vi "System Log.vi"(6 "VIs Hierarchy":i32, 8 "error in (no error)":errorcluster, 10 "Text to log":string, 11 "Object in":refnum<class>) -> (0 "error out":errorcluster)   [LabVIEW 2026, in "TALOS.lvlib"]
doc: "Log the text in the system log.\nVIs Hierarchy is used for selecting the name of which VI above this will be used in the log."
uses:
  TALOS.lvlib
  Ancestor/Ancestor/Ancestor.lvclass
  Ancestor/Ancestor/Ancestor.lvclass/Ancestor.ctl
  Classes/Log/Log.lvclass/Log.ctl
  Ancestor/Ancestor/Read ID.vi
  <vilib>/AdvancedString/Delimited String to 1D String Array.vi
  <vilib>/AdvancedString/Delimited String to 1D String Array (string).vi
  Classes/Log/Write.vi
  Generate Error.vi
  Date n Time.vi
  FGV/Error Memory/Get Error Description.vi
  Get PC name.vi
  <vilib>/Utility/error.llb/Clear Errors.vi
  FGV/Error Memory/Error Memory Core.vi
  Circus Root Path.vi
  FGV/Error Memory/Error Crt Lvl checker.vi
  FGV/Error Memory/Error Memory Core.vi/40c8088d-b597-4017-91af-faa98e00292e.vi
  FGV/Error Memory/Error Memory Core.vi/d4a3ab98-063c-4e44-b43d-fbdcfe6c2be2.vi
  <vilib>/Utility/LVClass/Get LV Class Name.vi
  Classes/Log/Rotate.vi
  Global Memory.vi
  Is in Packed Library.vi
  TALOS Root path.vi
  Read CSV worksheet.vi
  Global Constants.vi
  <vilib>/Utility/error.llb/General Error Handler.vi
  <vilib>/Comparison/Equal/Equal Functor/Equal Functor.lvclass
  Classes/Log/Log.lvclass
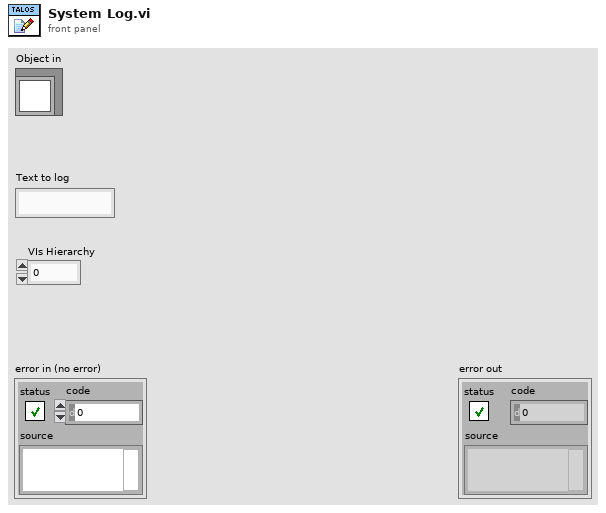
[diagram p1: front panel]
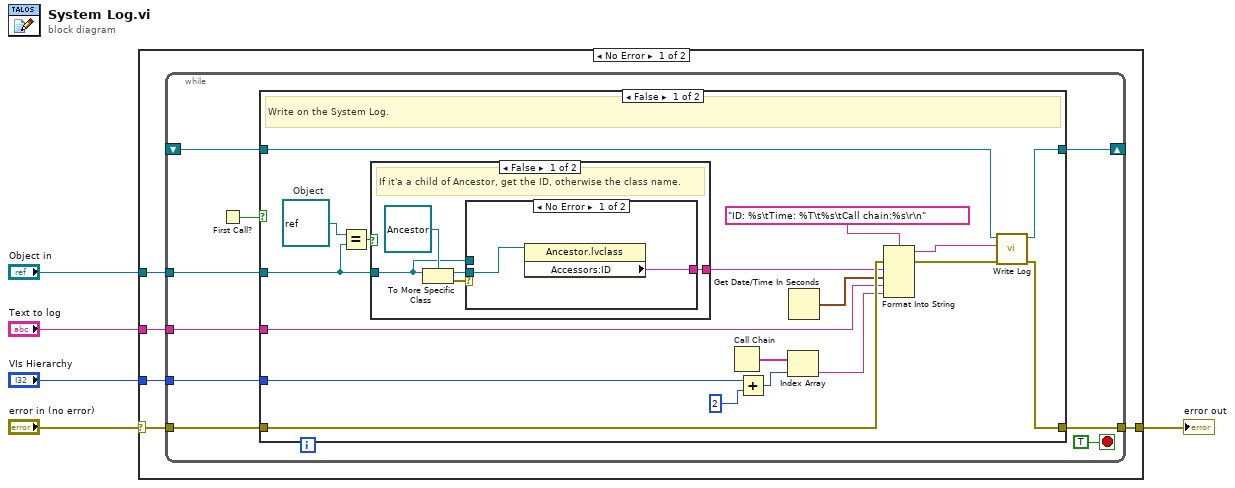
[diagram p0: block diagram]
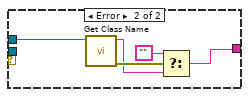
[diagram p2: hidden frame]
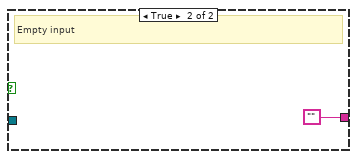
[diagram p3: hidden frame]
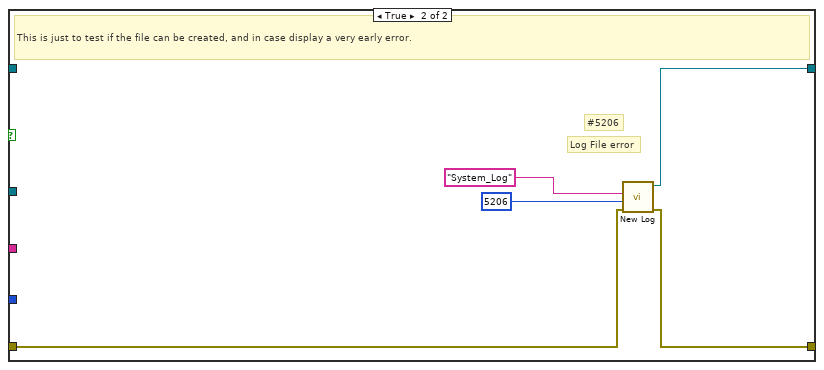
[diagram p4: hidden frame]
diagram:
  n1 = case shown="No Error" "error in (no error)" {
    selector: "error in (no error)" -> [w9 w56]
    tunnel: "Text to log" -> [w10 _]
    tunnel: "Object in" -> [w8 _]
    tunnel: [w7 w56] -> w2
    tunnel: "VIs Hierarchy" -> [w6 _]
    frame No Error {
      n2 = while {
        tunnel: w8 -> [w14]
        shift-right: [w17] -> _
        shift-left: _ -> [w16]
        tunnel: w10 -> [w15]
        tunnel: w9 -> [w13]
        tunnel: [w12] -> w7
        tunnel: w6 -> [w11]
        stop <- TRUE stop-if-true
        n3 = First Call?() -> (First Call?: T/F=w18:bool)
        n4 = case shown="False" w18 {
          tunnel: w14 -> [w23 _]
          tunnel: [w27 w51] -> w17
          tunnel: w16 -> [w26 _]
          tunnel: [w25 w52] -> w12
          tunnel: w15 -> [w31 _]
          tunnel: w13 -> [w37 w53]
          tunnel: w11 -> [w20 _]
          frame False {
            w24 = refnum<class> refnum  # Object
            # "Write on the System Log."
            n5 = Equal?(x=w24, y=w23) -> (x = y?=w22:bool)
            n6 = case shown="False" w22 {
              tunnel: [w42 ""] -> w33
              tunnel: w23 -> [w38 _]
              frame False {
                # "If it'a a child of Ancestor, get the ID, otherwise the class name."
                n7 = To More Specific Class(target class=refnum<class "Ancestor.lvclass"> refnum ("TALOS.lvlib:Ancestor.lvlib:Ancestor.lvclass"), reference=w38) -> (specific class reference=w40:refnum<class "Ancestor.lvclass">, error out=w39:errorcluster)  [unwired: 1 in]
                n8 = case shown="No Error" w39 {
                  tunnel: [w44 w46] -> w42
                  tunnel: w40 -> [w43 _]
                  tunnel: w38 -> [_ w49]
                  frame No Error {
                    n9 = property class="Ancestor.lvclass"(reference=w43) -> ("Accessors:ID"=w44:string)  [unwired: 1 in, 2 out]
                  }
                  frame Error {
                    n10 = call "Get Class Name.vi"("object"=w49) -> ("error out"=w48:errorcluster, "Class Name"=w47:string)  [unwired: 9 in]
                    n11 = Select(t="", s=w48, f=w47) -> (s? t:f=w46:string)
                  }
                }
              }
              frame True {
                # "Empty input"
              }
            }
            n12 = Call Chain() -> (call chain=w36:string[])
            n13 = Add(x=w20, y=2 ("index")) -> (x+y=w21:i32)
            n14 = Index Array(array=w36, index=w21) -> (element=w30:string)
            n15 = Get Date/Time In Seconds() -> (seconds since 1Jan1904=w32:timestamp)
            n16 = Format Into String(format string="ID: %s\tTime: %T\t%s\tCall chain:%s\r\n", error in=w37, w33, w32, w31, w30) -> (resulting string=w28:string, error out=w29:errorcluster)  [unwired: 1 in]
            n17 = call "Write Log.vi"("error in (no error)"=w29, "Text"=w28, "Log in"=w26) -> ("error out"=w25:errorcluster, "Log out"=w27:refnum<class "Log.lvclass">)  [unwired: 7 in]
          }
          frame True {
            # "Log File error"
            # "#5206"
            # "This is just to test if the file can be created, and in case display a very early error."
            n18 = call "New Log.vi"("error in (no error)"=w53, "Specific Error Code"=5206 ("Error Code"), "Name"="System_Log") -> ("error out"=w52:errorcluster, "Log out"=w51:refnum<class "Log.lvclass">)  [unwired: 7 in]
          }
        }
      }
    }
    frame Error {
    }
  }
  "error out" <- w2
